vi "Add Bricks.vi"(8 "error in (no error)":errorcluster, 10 "Piece Coordinates":T1[](array[typedef]), 11 "object in":refnum<class "Wall.lvclass">) -> (0 "error out":errorcluster, 3 "object out":refnum<class "Wall.lvclass">)   [LabVIEW 2017, in "Wall.lvclass"]
uses:
  Wall.lvclass
  Controls/Coordinates.ctl
  Wall.lvclass/Wall.ctl
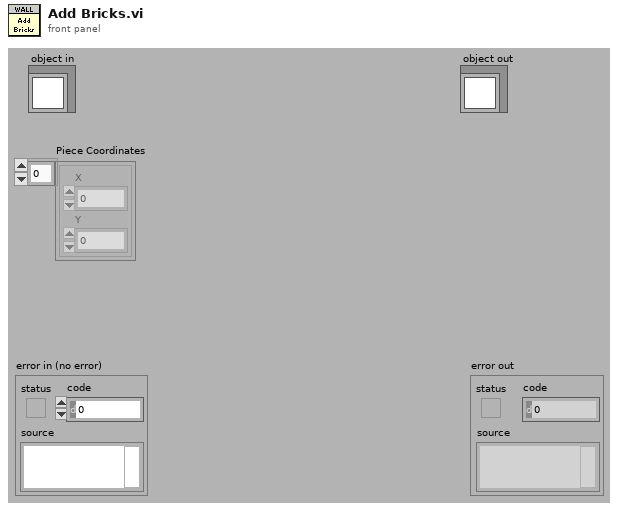
[diagram p1: front panel]
types:
  T1 = typedef "Coordinates.ctl" = cluster{"X":i32, "Y":i32}
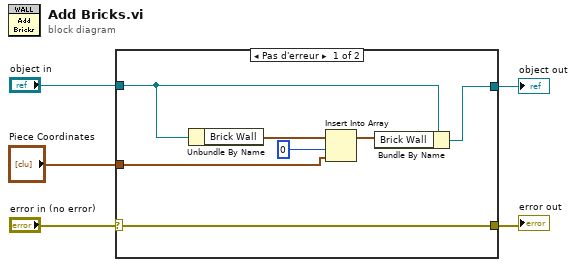
[diagram p0: block diagram]
diagram:
  n1 = case shown="Pas d'erreur" "error in (no error)" {
    selector: "error in (no error)" -> [w12 w14]
    tunnel: [w12 w14] -> w4
    tunnel: [w10 w13] -> w2
    tunnel: "object in" -> [w11 w13]
    tunnel: "Piece Coordinates" -> [w6 _]
    frame No Error {
      n2 = Unbundle By Name(w11) -> ("Brick Wall"=w9:T1[])
      n3 = Insert Into Array(array=w9, index=0 ("indice"), new element=w6) -> (w8:T1[])
      n4 = Bundle By Name(cluster=w11, "Brick Wall"=w8) -> (w10:refnum<class "Wall.lvclass">)
    }
    frame Error {
    }
  }
  "error out" <- w4
  "object out" <- w2
